vi "read status string.vi"() -> ()   [LabVIEW 2009]
panel:
  out "VISA resource name out":refnum<visa-resource-name>
  in  "VISA resource name":refnum<visa-resource-name>="GPIB0::12::INSTR"
  in  "error in (no error)":errorcluster
  out "read buffer":string
  in  "read? (f)":bool
  in  "bytes to read (1000)":u32=1000
  out "bytes read":u32
  out "error out":errorcluster
  in  "write buffer":string="RDPOW"
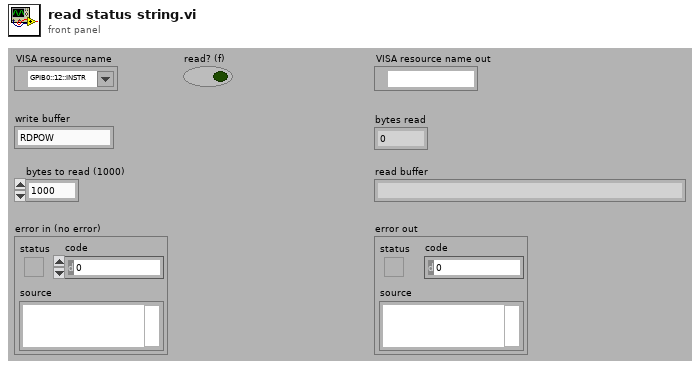
[diagram p1: front panel]
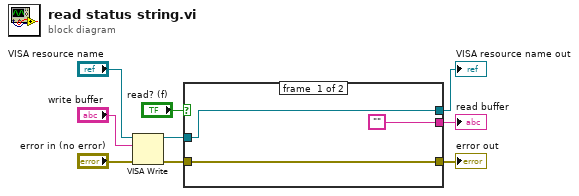
[diagram p0: block diagram]
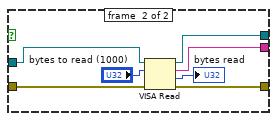
[diagram p2: hidden frame]
diagram:
  n1 = VISA Write(VISA resource name="VISA resource name", write buffer="write buffer", error in (no error)="error in (no error)") -> (VISA resource name out=w2:refnum<visa-resource-name>, error out=w1:errorcluster)  [unwired: 1 out]
  n2 = case shown="True" "read? (f)" {
    tunnel: w1 -> [w11 w13]
    tunnel: [w11 w19] -> w5
    tunnel: [w12 w17] -> w4
    tunnel: w2 -> [w12 w14]
    tunnel: ["" w16] -> w8
    frame #0 {
    }
    frame #1 {
      n3 = VISA Read(VISA resource name=w14, byte count="bytes to read (1000)", error in (no error)=w13) -> (VISA resource name out=w17:refnum<visa-resource-name>, read buffer=w16:string, return count=→"bytes read":u32, error out=w19:errorcluster)
    }
  }
  "error out" <- w5
  "read buffer" <- w8
  "VISA resource name out" <- w4
